vi "pr650_readbuffer.vi"(6 "error in (no error)":errorcluster, 7 "ref":refnum<vi>, 8 "reference":refnum<visa-resource-name>) -> (0 "error out":errorcluster, 1 "bytes at port":u32, 2 "return count":u32, 3 "read buffer":string, 4 "VISA resource name out":refnum<visa-resource-name>)   [LabVIEW 2010]
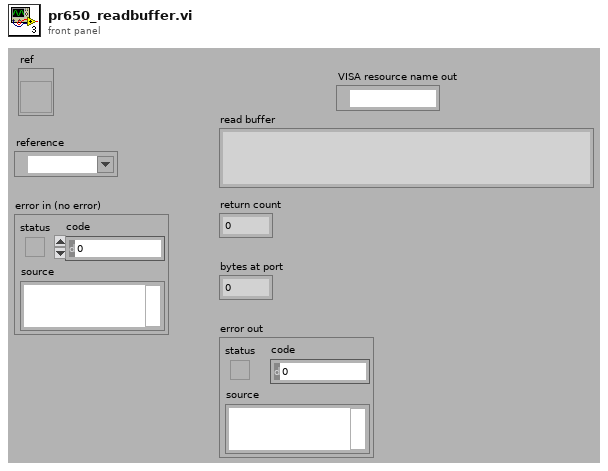
[diagram p1: front panel]
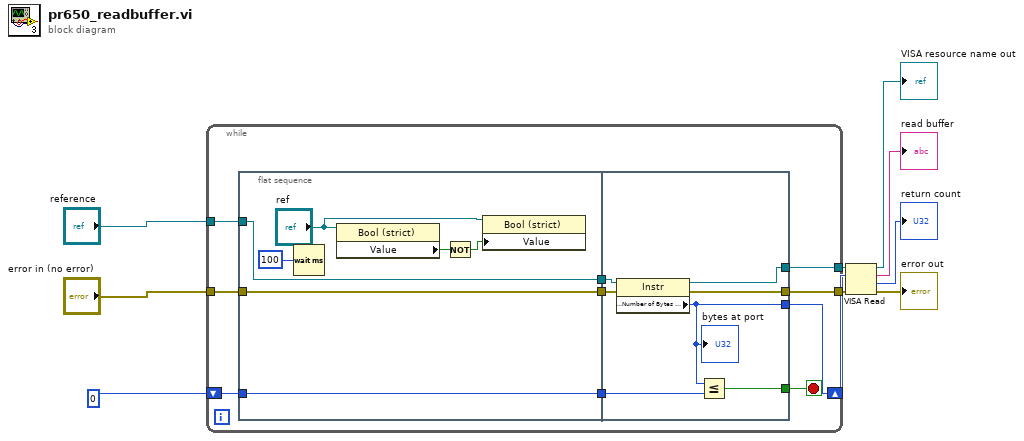
[diagram p0: block diagram]
diagram:
  n1 = while {
    tunnel: "reference" -> [w20]
    tunnel: [w19] -> w8
    tunnel: [w18] -> w7
    tunnel: "error in (no error)" -> [w17]
    shift-right: [w16] -> w1
    shift-left: u32 0 ("Bytes at Port") -> [w15]
    stop <- w14 stop-if-true
    n2 = flat-sequence {
      tunnel: w15 -> [w25]
      tunnel: w17 -> [w26]
      tunnel: w20 -> [w27]
      tunnel: [w27] -> w13
      tunnel: [w26] -> w12
      tunnel: [w25] -> w11
      tunnel: [w33] -> w19
      tunnel: [w32] -> w18
      tunnel: [w30] -> w16
      tunnel: [w28] -> w14
      tunnel: w13 -> [w34]
      tunnel: w12 -> [w31]
      tunnel: w11 -> [w29]
      frame #0 {
        n3 = Wait (ms)(milliseconds to wait=u32 100) -> ()  [unwired: 1 out]
        n4 = property class="Bool (strict)"(reference="ref") -> ("Value"=w23:bool)  [unwired: 1 in, 2 out]
        n5 = Not(x=w23) -> (.not. x?=w22:bool)
        n6 = property class="Bool (strict)"(reference="ref", "Value"=w22) -> ()  [unwired: 1 in, 2 out]
      }
      frame #1 {
        n7 = property class="Instr"(reference=w34, error in=w31) -> (reference out=w33:refnum<visa-resource-name>, error out=w32:errorcluster, "Serial Settings:Number of Bytes at Serial Port"=w30:u32)
        "bytes at port" <- w30
        n8 = Less Or Equal?(x=w30, y=w29) -> (x <= y?=w28:bool)
      }
    }
  }
  n9 = VISA Read(VISA resource name=w8, byte count=w1, error in (no error)=w7) -> (VISA resource name out=→"VISA resource name out":refnum<visa-resource-name>, read buffer=→"read buffer":string, return count=→"return count":u32, error out=→"error out":errorcluster)
